vi "Module Name--constant.vi"() -> (3 "Module Name":string)   [LabVIEW 2024, in "DQMH Power Requests.lvlib"]
doc: "Return the name of the module that owns this VI. \n_____\nBased on Delacor QMH Project Template 4.2.1.64."
uses:
  DQMH Power Requests.lvlib
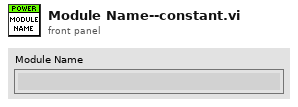
[diagram p1: front panel]
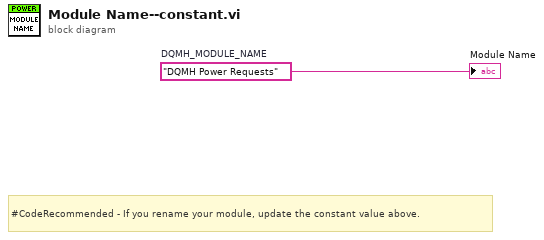
[diagram p0: block diagram]
diagram:
  w1 = "DQMH Power Requests"  # DQMH_MODULE_NAME
  # "#CodeRecommended - If you rename your module, update the constant value above."
  "Module Name" <- w1
